vi "GT_SetSoftLimit.vi"(6 "negative":i32, 7 "positive":i32, 10 "axis":i16, 11 "rtn_In":cluster{"rtn":i16, "Func":string}) -> (2 "axis":i16, 3 "rtn_out":cluster{"rtn":i16, "Func":string})   [LabVIEW 2014]
uses:
  VC6/gts.dll
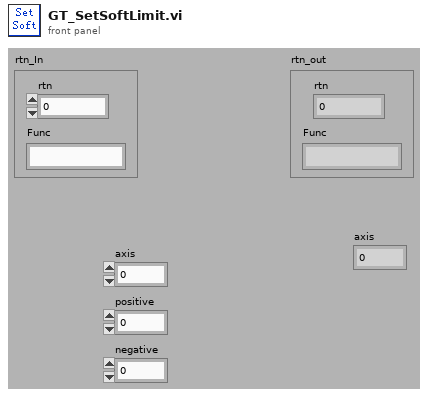
[diagram p1: front panel]
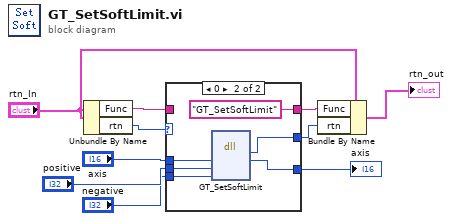
[diagram p0: block diagram]
diagram:
  n1 = Unbundle By Name("rtn_In") -> ("Func"=w3:string, "rtn"=w6:i16)
  n2 = case shown="0" w6 {
    selector: w6 -> [w13 _]
    tunnel: "axis" -> [w12 w19]
    tunnel: "positive" -> [_ w18]
    tunnel: "negative" -> [_ w17]
    tunnel: [w13 w16] -> w5
    tunnel: [w12 w15] -> w7
    tunnel: [w11 "GT_SetSoftLimit" ("Func")] -> w4
    tunnel: w3 -> [w11 _]
    frame Default {
    }
    frame 0 {
      n3 = dll-call lib="PTH2Fabs DNewGTS AC-800LWin7版源程序-20170926gts85VC6gts.dll" fn="GT_SetSoftLimit"("axis"=w19, "positive"=w18, "negative"=w17) -> ("rtn"=w16:i16, "axis"=w15:i16)  [unwired: 5 in, 2 out]
    }
  }
  "axis" <- w7
  n4 = Bundle By Name(cluster="rtn_In", "Func"=w4, "rtn"=w5) -> (→"rtn_out":cluster{"rtn":i16, "Func":string})
